vi "Graphics-Set Plot Properties.vi"(0 "Plot in":refnum<vi>, 7 "properties":T1, 11 "error in (no error)":errorcluster) -> (4 "Plot out":refnum<vi>, 15 "error out":errorcluster)   [LabVIEW 2020]
uses:
  Graphics-Plot Properties.ctl
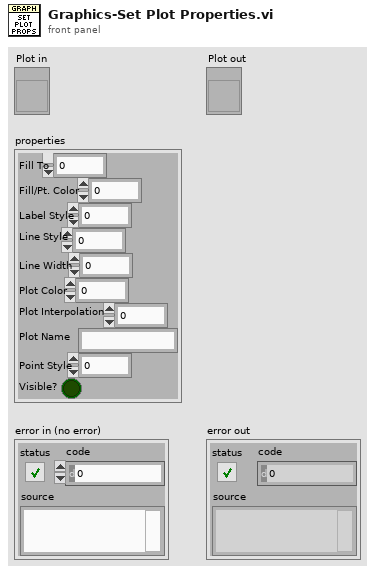
[diagram p1: front panel]
types:
  T1 = typedef "Graphics-Plot Properties.ctl" = cluster{"Fill To":i16, "Fill/Pt. Color":u32, "Label Style":u8, "Line Style":u8, "Line Width":u8, "Plot Color":u32, "Plot Interpolation":u8, "Plot Name":string, "Point Style":u8, "Visible?":bool}
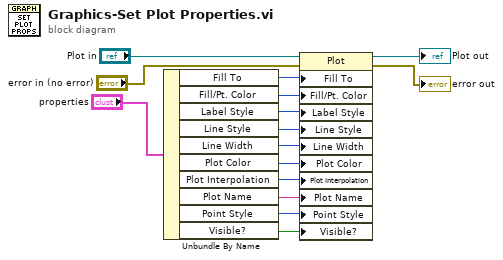
[diagram p0: block diagram]
diagram:
  n1 = Unbundle By Name("properties") -> ("Fill To"=w10:i16, "Fill/Pt. Color"=w9:u32, "Label Style"=w8:u8, "Line Style"=w7:u8, "Line Width"=w6:u8, "Plot Color"=w5:u32, "Plot Interpolation"=w4:u8, "Plot Name"=w3:string, "Point Style"=w2:u8, "Visible?"=w1:bool)
  n2 = property class="Plot"(reference="Plot in", error in="error in (no error)", "Fill To"=w10, "Fill/Pt. Color"=w9, "Label Style"=w8, "Line Style"=w7, "Line Width"=w6, "Plot Color"=w5, "Plot Interpolation"=w4, "Plot Name"=w3, "Point Style"=w2, "Visible?"=w1) -> (reference out=→"Plot out":refnum<vi>, error out=→"error out":errorcluster)
